vi "Build Multiplot XY Graph.vi"(8 "error in (no error)":errorcluster, 9 "FGV Build Multiplot XY":T1, 10 "Sensor Array in":dbl[](array[numeric]), 11 "Time":dbl) -> (0 "error out":errorcluster, 3 "Multiplot XY Array":cluster{dbl[], dbl[]}[](array[cluster]))   [LabVIEW 2021]
uses:
  FGV Multiplot Action.ctl
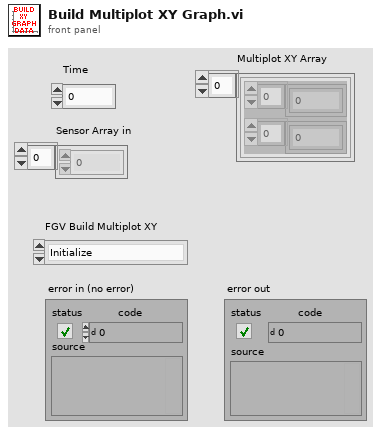
[diagram p1: front panel]
types:
  T1 = typedef "FGV Multiplot Action.ctl" = enum16{"Initialize", "Read"}
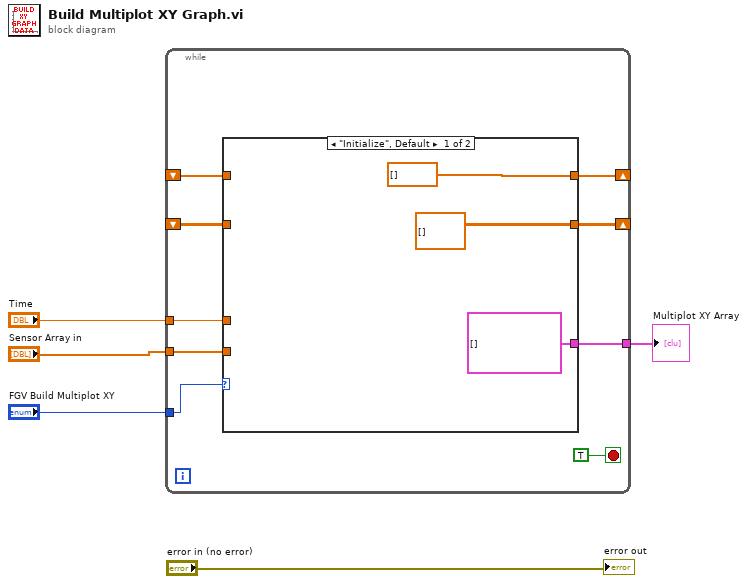
[diagram p0: block diagram]
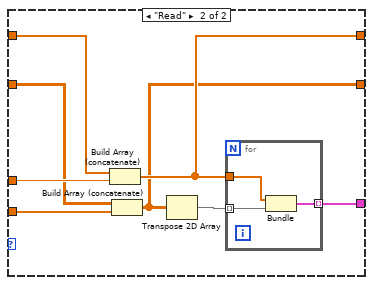
[diagram p2: hidden frame]
diagram:
  n1 = while {
    tunnel: "Time" -> [w14]
    tunnel: [w13] -> w4
    tunnel: "Sensor Array in" -> [w12]
    shift-right: [w10] -> _
    shift-left: _ -> [w9]
    shift-right: [w8] -> _
    shift-left: _ -> [w7]
    tunnel: "FGV Build Multiplot XY" -> [w6]
    stop <- TRUE stop-if-true
    n2 = case shown="\"Initialize\", Default" w6 {
      tunnel: w14 -> [_ w25]
      tunnel: [cluster{dbl[], dbl[]}[] [] w24] -> w13
      tunnel: w12 -> [_ w23]
      tunnel: [dbl[] [] w21] -> w10
      tunnel: w9 -> [_ w20]
      tunnel: [dbl[][] [] w19] -> w8
      tunnel: w7 -> [_ w18]
      frame "Initialize", Default {
      }
      frame "Read" {
        n3 = Build Array (concatenate)(w20, w25) -> (w21:dbl[])
        n4 = Build Array (concatenate)(w18, w23) -> (w19:dbl[][])
        n5 = Transpose 2D Array(2D array=w19) -> (transposed array=w22:dbl[][])
        n6 = for {
          tunnel: w22 -> [w28] mode=indexing
          tunnel: w21 -> [w27]
          tunnel: [w26] -> w24 mode=indexing
          n7 = Bundle(w27, w28) -> (w26:cluster{dbl[], dbl[]})  [unwired: 1 in]
        }
      }
    }
  }
  "Multiplot XY Array" <- w4
  "error out" <- "error in (no error)"
